vi "GetText.vi"(8 "error in":errorcluster, 11 "node in":refnum<class "CEF_serializable node folder.lvclass">) -> (0 "error out":errorcluster, 1 "additional text":string, 2 "text":string, 3 "node out":refnum<class "CEF_serializable node folder.lvclass">, 4 "glyph":string)   [LabVIEW 2023, in "CEF_serializable node folder.lvclass"]
doc: "Returns the text representation of the node used for the tree control.Copyright 2017 National Instruments Corporation\n\nLicensed under the Apache License, Version 2.0 (the \"License\"); you may not use this file except in compliance with the License. You may obtain a copy of the License at http://www.apache.org/licenses/LICENSE-2.0\nUnless required by applicable law or agreed to in writing, software distributed under the License is distributed on an \"AS IS\" BASIS, WITHOUT WARRANTIES OR CONDITIONS OF ANY KIND, either express or implied. See the License for the specific language governing permissions and limitations under the License."
uses:
  CEF_serializable node folder.lvclass
  serializable node/NISE_CEF_serializable node.lvclass
  CEF_serializable node folder.lvclass/CEF_serializable node folder.ctl
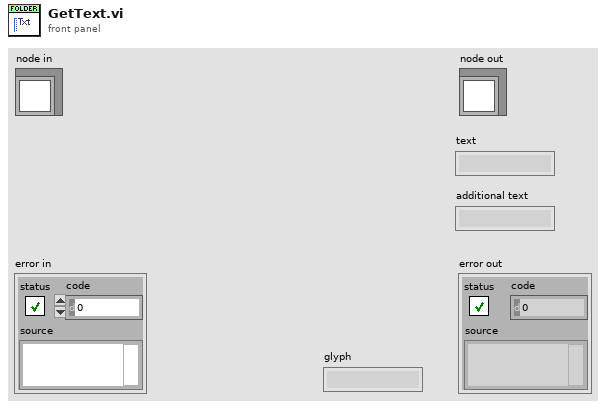
[diagram p1: front panel]
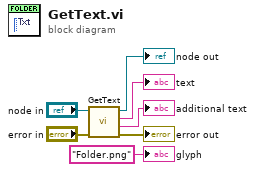
[diagram p0: block diagram]
diagram:
  n1 = call-parent "GetText.vi"("error in"="error in", "node in"="node in") -> ("error out"=→"error out":errorcluster, "additional text"=→"additional text":string, "text"=→"text":string, "node out"=→"node out":refnum<class "CEF_serializable node folder.lvclass">)  [unwired: 5 in, 1 out]
  "glyph" <- "Folder.png" ("glyph")
